vi "Greyscale Image Averager3.vi"(0 "Img Array IN":T1[](array[typedef]), 7 "Image Dst In":T1, 9 "usb":bool, 11 "error in (no error)":errorcluster) -> (4 "Img Array Out":T1[](array[typedef]), 8 "Image Dst Out":T1, 15 "error out":errorcluster)   [LabVIEW 2013]
doc: "Calculate an averaged image from an array of images."
uses:
  <vilib>/vision/Image Controls.llb/IMAQ Image.ctl
panel:
  in  "Viewer":bool
  out "Numeric":i32
  out "Image":T1(plugin-control)
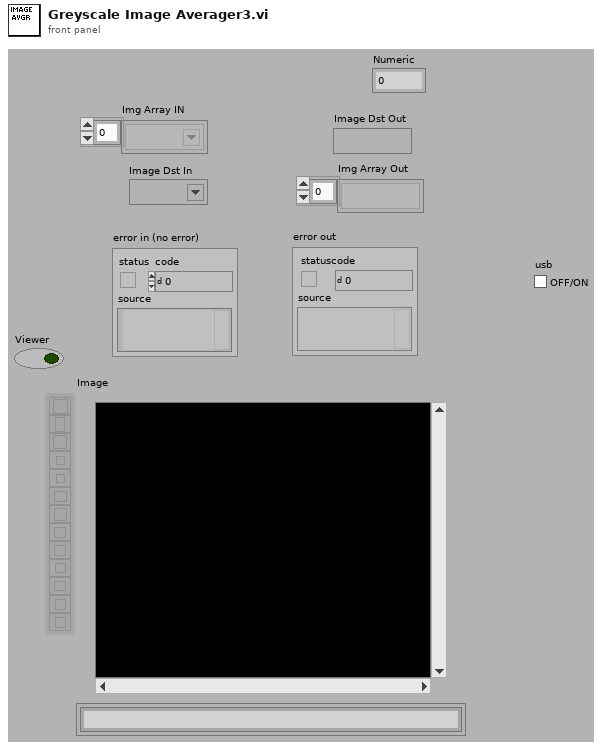
[diagram p1: front panel]
types:
  T1 = typedef "IMAQ Image.ctl" = refnum<image>
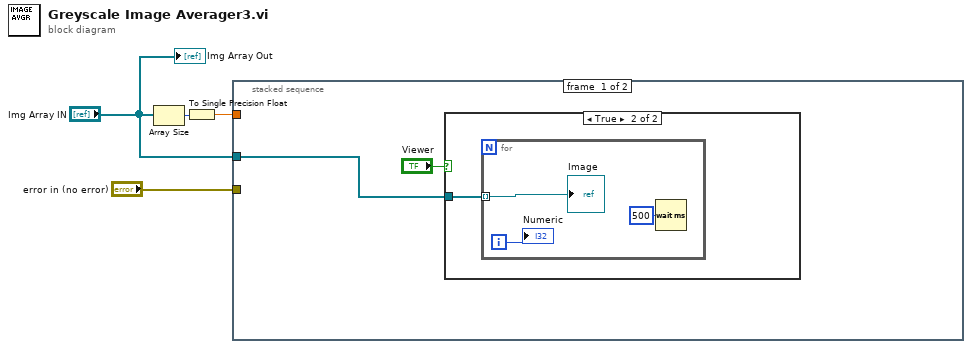
[diagram p0: block diagram]
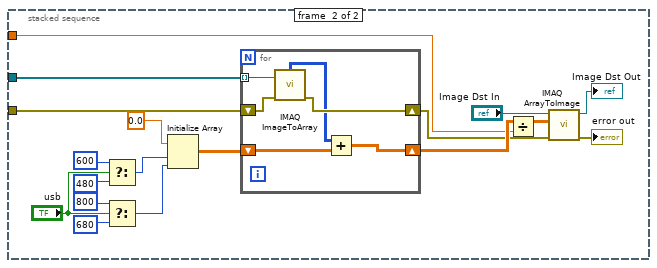
[diagram p3: hidden frame]
diagram:
  n1 = Array Size(array="Img Array IN") -> (size(s)=w4:i32)
  n2 = To Single Precision Float(number=w4) -> (single precision float=w3:sgl)
  n3 = stacked-sequence {
    tunnel: w3 -> [_ w23]
    tunnel: "Img Array IN" -> [w6 w28]
    tunnel: "error in (no error)" -> [_ w27]
    frame #0 {
      n4 = case shown="True" "Viewer" {
        tunnel: w6 -> [_ w7]
        frame False {
        }
        frame True {
          n5 = for {
            tunnel: w7 -> [w10] mode=indexing
            i -> [w9]
            n6 = Wait (ms)(milliseconds to wait=u32 500 ("millisecond timer value")) -> ()  [unwired: 1 out]
            "Image" <- w10
            "Numeric" <- w9
          }
        }
      }
    }
    frame #1 {
      n7 = Select(t=600 ("dimension size"), s="usb", f=480 ("dimension size")) -> (s? t:f=w12:i32)
      n8 = Select(t=800 ("dimension size"), s="usb", f=680 ("dimension size")) -> (s? t:f=w11:i32)
      n9 = Initialize Array(0.0, w12, w11) -> (w25:dbl[][])
      n10 = for {
        tunnel: w28 -> [w34] mode=indexing
        shift-right: [w32] -> w19
        shift-left: w27 -> [w33]
        shift-right: [w30] -> w24
        shift-left: w25 -> [w31]
        n11 = call "IMAQ ImageToArray"("error in (no error)"=w33, "Image"=w34) -> ("error out"=w32:errorcluster, "Image Pixels (U8)"=w29:u8[][])  [unwired: 2 in, 3 out]
        n12 = Add(x=w29, y=w31) -> (x+y=w30:dbl[][])
      }
      n13 = Divide(x=w24, y=w23) -> (x/y=w21:dbl[][])
      n14 = call "IMAQ ArrayToImage"("error in (no error)"=w19, "Image Pixels (U8)"=w21, "Image"="Image Dst In") -> ("error out"=→"error out":errorcluster, "Image Out"=→"Image Dst Out":T1)  [unwired: 7 in]
    }
  }
  "Img Array Out" <- "Img Array IN"
